vi "niDTS BT INSTR TX Configure.vi"(6 "Ports":string[](array[string]), 8 "error in (no error)":errorcluster, 10 "Expected Power From DUT":dbl format="%#_13g", 11 "niDTS BT INSTR TX in":refnum<class "niDTS BT INSTR TX.lvclass">) -> (0 "error out":errorcluster, 3 "niDTS BT INSTR TX out":refnum<class "niDTS BT INSTR TX.lvclass">)   [LabVIEW 2015, in "niDTS BT.lvlib" / "niDTS BT INSTR TX.lvclass"]
uses:
  niDTS BT INSTR TX.lvclass
  niDTS BT INSTR TX.lvclass/niDTS BT INSTR TX.ctl
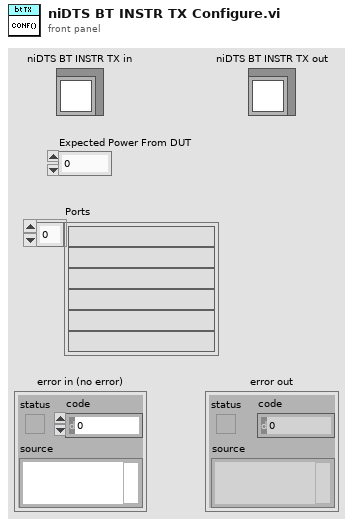
[diagram p1: front panel]
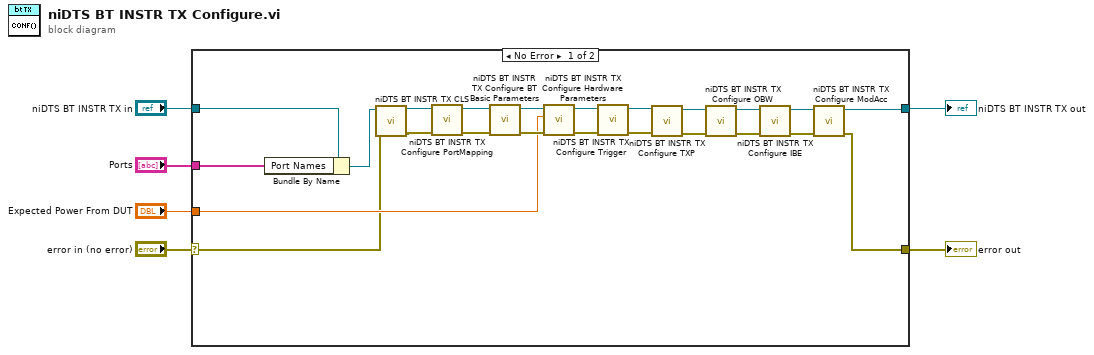
[diagram p0: block diagram]
diagram:
  n1 = case shown="No Error" "error in (no error)" {
    selector: "error in (no error)" -> [w8 w31]
    tunnel: [w17 w31] -> w5
    tunnel: [w16 w30] -> w3
    tunnel: "niDTS BT INSTR TX in" -> [w15 w30]
    tunnel: "Ports" -> [w14 _]
    tunnel: "Expected Power From DUT" -> [w13 _]
    frame No Error {
      n2 = Bundle By Name(cluster=w15, "Port Names"=w14) -> (w9:refnum<class "niDTS BT INSTR TX.lvclass">)
      n3 = call-dynamic "niDTS BT INSTR TX CLS.vi"("error in (no error)"=w8, "niDTS BT INSTR TX in"=w9) -> ("error out"=w7:errorcluster, "niDTS BT INSTR TX out"=w10:refnum<class "niDTS BT INSTR TX.lvclass">)  [unwired: 8 in]
      n4 = call-dynamic "niDTS BT INSTR TX Configure PortMapping.vi"("error in (no error)"=w7, "niDTS BT INSTR TX in"=w10) -> ("error out"=w11:errorcluster, "niDTS BT INSTR TX out"=w12:refnum<class "niDTS BT INSTR TX.lvclass">)  [unwired: 8 in]
      n5 = call-dynamic "niDTS BT INSTR TX Configure BT Basic Parameters.vi"("error in (no error)"=w11, "niDTS BT INSTR TX in"=w12) -> ("error out"=w27:errorcluster, "niDTS BT INSTR TX out"=w29:refnum<class "niDTS BT INSTR TX.lvclass">)  [unwired: 8 in]
      n6 = call-dynamic "niDTS BT INSTR TX Configure Hardware Parameters.vi"("error in (no error)"=w27, "MaxInputPower"=w13, "niDTS BT INSTR TX in"=w29) -> ("error out"=w26:errorcluster, "niDTS BT INSTR TX out"=w28:refnum<class "niDTS BT INSTR TX.lvclass">)  [unwired: 7 in]
      n7 = call "niDTS BT INSTR TX Configure Trigger.vi"("error in (no error)"=w26, "niDTS BT INSTR TX in"=w28) -> ("error out"=w25:errorcluster, "niDTS BT INSTR TX out"=w24:refnum<class "niDTS BT INSTR TX.lvclass">)  [unwired: 8 in]
      n8 = call "niDTS BT INSTR TX Configure TXP.vi"("error in (no error)"=w25, "niDTS BT INSTR TX in"=w24) -> ("error out"=w23:errorcluster, "niDTS BT INSTR TX out"=w22:refnum<class "niDTS BT INSTR TX.lvclass">)  [unwired: 8 in]
      n9 = call "niDTS BT INSTR TX Configure OBW.vi"("error in (no error)"=w23, "niDTS BT INSTR TX in"=w22) -> ("error out"=w20:errorcluster, "niDTS BT INSTR TX out"=w21:refnum<class "niDTS BT INSTR TX.lvclass">)  [unwired: 8 in]
      n10 = call "niDTS BT INSTR TX Configure IBE.vi"("error in (no error)"=w20, "niDTS BT INSTR TX in"=w21) -> ("error out"=w18:errorcluster, "niDTS BT INSTR TX out"=w19:refnum<class "niDTS BT INSTR TX.lvclass">)  [unwired: 8 in]
      n11 = call "niDTS BT INSTR TX Configure ModAcc.vi"("error in (no error)"=w18, "niDTS BT INSTR TX in"=w19) -> ("error out"=w17:errorcluster, "niDTS BT INSTR TX out"=w16:refnum<class "niDTS BT INSTR TX.lvclass">)  [unwired: 8 in]
    }
    frame Error {
    }
  }
  "error out" <- w5
  "niDTS BT INSTR TX out" <- w3
